vi "203_SubscribePoll_NonStreamingNode.vi"() -> ()   [LabVIEW 2009]
uses:
  <instrlib>/Zurich Instruments LabOne/Public/Data/ziTypeDoubleDataTS.ctl
  <instrlib>/Zurich Instruments LabOne/Public/Configure/ziGetValueString.vi
  <instrlib>/Zurich Instruments LabOne/Public/Data/ziGetEventDoubleDataTS.vi
  <instrlib>/Zurich Instruments LabOne/Zurich Instruments LabOne.lvlib
panel:
  out "Tab Control":T1(tab)
  out "Value Double":dbl
  out "Waveform Chart HF2":dbl(graph)
  out "Waveform Chart":dbl[](graph)
  out "Sample Out":T2
  in  "stop":bool
  out "Connected?":bool
  out "Error Out":errorcluster
  in  "Address":string="DEV"
  # "Subscribe and Poll \nnonstreaming Node \nThis VI shows how to subscribe and poll data from a nonstreaming node.\n\n\nSee block diagram for the VI description.\n\nRequirements: Any Zurich Instrument Product\n\nTo run\n1. Type the Instrument ID \n2. Run the VI\n3. Change the signal output offset value in the LabOne GUI. This will trigger a poll for this value and update the waveform chart. \n\nTested Devices:\n- HF2LI\n- UHFLI\n- MFLI\n\n(c) Zurich Instruments.  ALL RIGHTS RESERVED."
  # "Test how the poll works by changing a value in the LabOne GUI\n1- Run the VI. \n2- On the LabOne GUI change the signal output values (as indicated on the right) and see that the values updated in the waveform chart.  \n\nThe signal output panel might slightly differ depending on the instrument and installed options"
  # "The data server that handles communication with HF2 Instruments, ziServer. exe, for non-streaming nodes provides only the  the values, which could be doubles or integers. In this example, we subscribe to sigouts/0/offset, which is a double.  \n\nThe values in the subscribed node are only polled when there is a change in the values. Therefore, to update the waveform chart in this example, you can update the value in the GUI.  \n\nNote that the streaming nodes, such as demod nodes, are returned with their timestamps."
  # "Polling from a node \nThe samples from each node come with a value and a timestamp. This is returned as a cluster with the ziGetEvet VI.  \n\nThe values in the subscribed node are only polled when there is a change in the values. Therefore, to update the waveform chart in this example, you can update the value in the GUI."
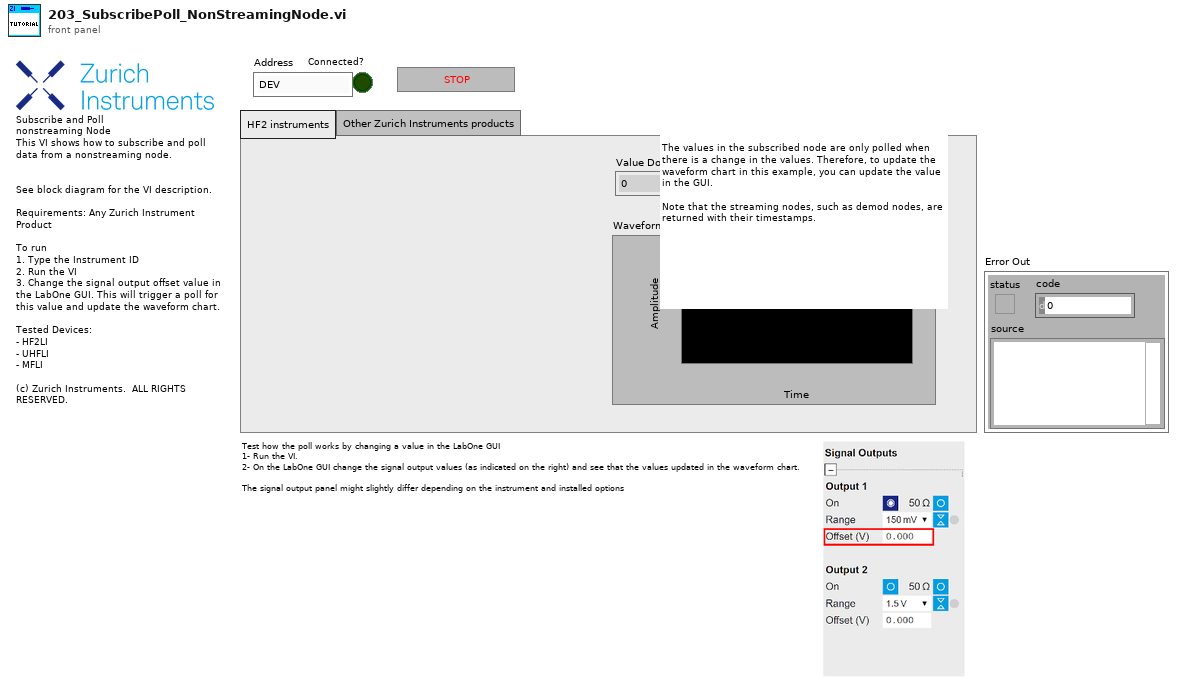
[diagram p1: front panel]
types:
  T1 = enum32{"HF2 instruments", "Other Zurich Instruments products"}
  T2 = typedef "Zurich Instruments LabOne.lvlib/ziTypeDoubleDataTS.ctl" = cluster{"Timestamp (ticks)":u64[], "Value":dbl[]}
  T3 = typedef "Zurich Instruments LabOne.lvlib/ziTypeHandle.ctl" = cluster{"handleValid":bool, "Conn":u64, "Path Prefix":string, "Handle":u64, "Connected":bool, "Clockbase(s)":dbl}
  T4 = typedef "Zurich Instruments LabOne.lvlib/ziTypePollType.ctl" = enum16{"NONE", "DOUBLE_DATA", "INTEGER_DATA", "DEMOD_SAMPLE", "SCOPE_WAVE_HF2", "AUXIN_SAMPLE", "DIO_SAMPLE", "BYTE_ARRAY", "PWA_WAVE", "9", "10", "11", "12", "13", "14", "15", "TREE_CHANGE_DEPRI", "17", "ERROR", "19", "20", "21", "22", "23", "24", "25", "26", "27", "28", "29", "30", "31", "DOUBLE_DATA_TS", "INTEGER_DATA_TS", "34", "SCOPE_WAVE", "SCOPE_WAVE_EX", "37", "BYTE_ARRAY_TS", "39", "40", "41", "42", "43", "44", "45", "CNT_DATA", "47", "TREE_CHANGE", "49", "50", "51", "52", "53", "54", "55", "56", "57", "58", "59", "60", "61", "62", "63", "SWEEPER_DATA", "SPECTRUM_DATA", "ADVISOR_DATA", "VECTOR_DATA", "IMP_DATA"}
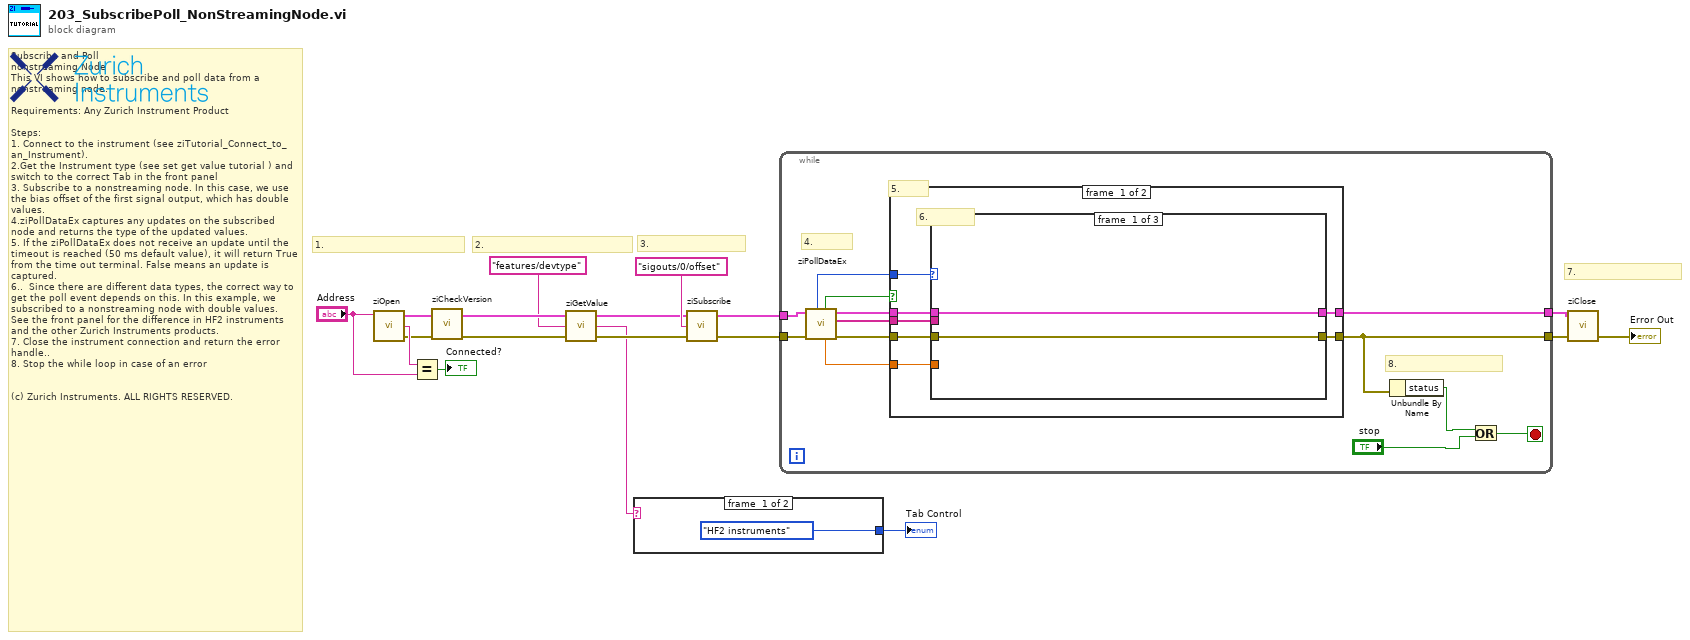
[diagram p0: block diagram]
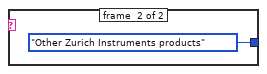
[diagram p2: hidden frame]
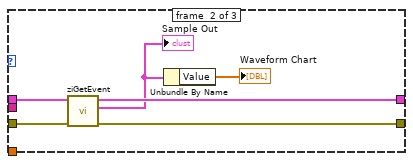
[diagram p3: hidden frame]
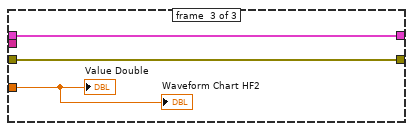
[diagram p4: hidden frame]
diagram:
  # "3."
  # "2."
  # "1."
  # "7."
  # "Subscribe and Poll \nnonstreaming Node \nThis VI shows how to subscribe and poll data from a nonstreaming node. \n\nRequirements: Any Zurich Instrument Product\n\nSteps:\n1. Connect to the instrument (see ziTutorial_Connect_to_an_Instrument).\n2.Get the Instrument type (see set get value tutorial ) and switch to the correct Tab in the front panel\n3. Subscribe to a nonstreaming node. In this case, we use the bias offset of the first signal output, which has double values.\n4.ziPollDataEx captures any updates on the subscribed node and returns the type of the updated values. \n5. If the ziPollDataEx does not receive an update until the timeout is reached (50 ms default value), it will return True from the time out terminal. False means an update is captured.\n6..  Since there are different data types, the correct way to get the poll event depends on this. In this example, we subscribed to a nonstreaming node with double values.  See the front panel for the difference in HF2 instruments and the other Zurich Instruments products. \n7. Close the instrument connection and return the error handle..\n8. Stop the while loop in case of an error\n\n\n(c) Zurich Instruments. ALL RIGHTS RESERVED."
  n1 = call <instrlib>:"ziOpen.vi"("Address"="Address") -> ("Error Out"=w13:errorcluster, "Selected Device"=w16:string, "HandleOut"=w14:T3)  [unwired: 1 in, 2 out]
  n2 = Equal?(x=w16, y="Address") -> (x = y?=→"Connected?":bool)
  n3 = call <instrlib>:"ziCheckVersion.vi"("Handle In"=w14, "Error In"=w13) -> ("Handle Out"=w6:T3, "Error Out"=w7:errorcluster)  [unwired: 11 in, 1 out]
  n4 = call-poly <instrlib>:"ziGetValue.vi"("error in"=w7, "Path"="features/devtype", "Handle In"=w6) -> ("error out"=w3:errorcluster, "Value"=w1:string, "Handle Out"=w2:T3)
  n5 = case shown="Default" w1 {
    tunnel: [T1."HF2 instruments" ("Tab Control") T1."Other Zurich Instruments products" ("Tab Control")] -> w4
    frame #0 {
    }
    frame #1 {
    }
  }
  "Tab Control" <- w4
  n6 = call <instrlib>:"ziSubscribe.vi"("error in"=w3, "Path ()"="sigouts/0/offset" ("path"), "Handle In"=w2) -> ("error out"=w11:errorcluster, "Handle Out"=w10:T3)  [unwired: 1 in]
  n7 = while {
    tunnel: w11 -> [w31]
    tunnel: w10 -> [w32]
    tunnel: [w33] -> w9
    tunnel: [w24] -> w8
    stop <- w21 stop-if-true
    # "8."
    # "5."
    # "4."
    n8 = call <instrlib>:"ziPollDataEx.vi"("error in"=w31, "Handle In"=w32) -> ("error out"=w29:errorcluster, "PathArray"=w26:string[], "Handle Out"=w30:T3, "Value Double"=w25:dbl, "Timed Out"=w28:bool, "ziValueType"=w27:T4)  [unwired: 2 in, 2 out]
    n9 = case shown="False" w28 {
      tunnel: [w40 w53] -> w33
      tunnel: [w39 w52] -> w24
      tunnel: w30 -> [w38 w53]
      tunnel: w29 -> [w37 w52]
      tunnel: w27 -> [w36 _]
      tunnel: w26 -> [w35 _]
      tunnel: w25 -> [w34 _]
      frame #0 {
        # "6."
        n10 = case shown="\"DOUBLE_DATA_TS\"" w36 {
          tunnel: [w42 w48 w51] -> w40
          tunnel: [w41 w43 w50] -> w39
          tunnel: w38 -> [w42 w47 w51]
          tunnel: w37 -> [w41 w46 w50]
          tunnel: w35 -> [_ _ _]
          tunnel: w34 -> [_ _ w49]
          frame #0 {
          }
          frame #1 {
            n11 = call-poly <instrlib>:"ziGetEvent.vi"("Error In"=w46, "Handle In"=w47) -> ("Error Out"=w43:errorcluster, "Sample Out"=w44:T2, "Handle Out"=w48:T3)  [unwired: 7 in]
            "Sample Out" <- w44
            n12 = Unbundle By Name(w44) -> ("Value"=→"Waveform Chart":dbl[])
          }
          frame #2 {
            "Value Double" <- w49
            "Waveform Chart HF2" <- w49
          }
        }
      }
      frame #1 {
      }
    }
    n13 = Unbundle By Name(w24) -> ("status"=w23:bool)
    n14 = Or(x=w23, y="stop") -> (x .or. y?=w21:bool)
  }
  n15 = call <instrlib>:"ziClose.vi"("Error In"=w8, "Handle In"=w9) -> ("Error Out"=→"Error Out":errorcluster)  [unwired: 2 in, 1 out]
